vi "Error Handler Main.vi"(8 "Error In":errorcluster) -> ()   [LabVIEW 2014]
uses:
  <vilib>/Platform/TimedLoop/XDataNode/timing_clust.ctl
  <vilib>/Platform/TimedLoop/XDataNode/nitl_modes.ctl
  <vilib>/Platform/TimedLoop/XDataNode/wakeup.ctl
  <vilib>/Utility/error.llb/DialogType.ctl
  Stop Button/SubVI/Get Stop Button Status.vi
  <vilib>/platform/TimedLoop/XDataNode/XDataNode.xnode
  <vilib>/Platform/TimedLoop/XDataNode/XDNodeRunTimeDep.lvlib
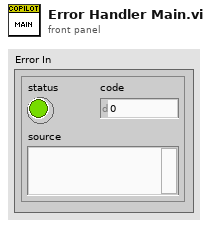
[diagram p1: front panel]
types:
  T1 = typedef "XDNodeRunTimeDep.lvlib/timing_clust.ctl" = cluster{"Expected End [f-1]":u64, "Actual End [f-1]":u64, "Finished Late? [f-1]":bool, "Expected End [i-1]":u64, "Actual End [i-1]":u64, "Finished Late? [i-1]":bool, "Expected Start [i]":u64, "Actual Start [i]":u64, "Expected Start [f]":u64, "Actual Start [f]":u64, "Source Name":string, "Structure Name":string, "Period":i64, "Deadline":i64, "Offset":i64, "Start":i64, "Priority":i32, "Timeout":i32, "Mode":T2, "Wakeup Reason":T3, "Error":errorcluster, "Source Type":string, "Secondary Source Type":string, "Global End Time":u64, "Global Start Time":u64, "Frame Duration":u64, "Iteration Duration":u64, "Assigned CPU":i32, "I/O Scan Engine Mode":u32}
  T2 = typedef "XDNodeRunTimeDep.lvlib/nitl_modes.ctl" = enum32{"No Change", "Process missed periods, maintain original phase", "Discard missed periods, maintain original phase", "Process missed periods, ignore original phase", "Discard missed periods, ignore original phase"}
  T3 = typedef "XDNodeRunTimeDep.lvlib/wakeup.ctl" = enum32{"Normal", "Aborted", "Asynchronous wakeup", "Timing source error", "Timed loop error", "Timeout"}
  T4 = typedef "DialogType.ctl" = u16
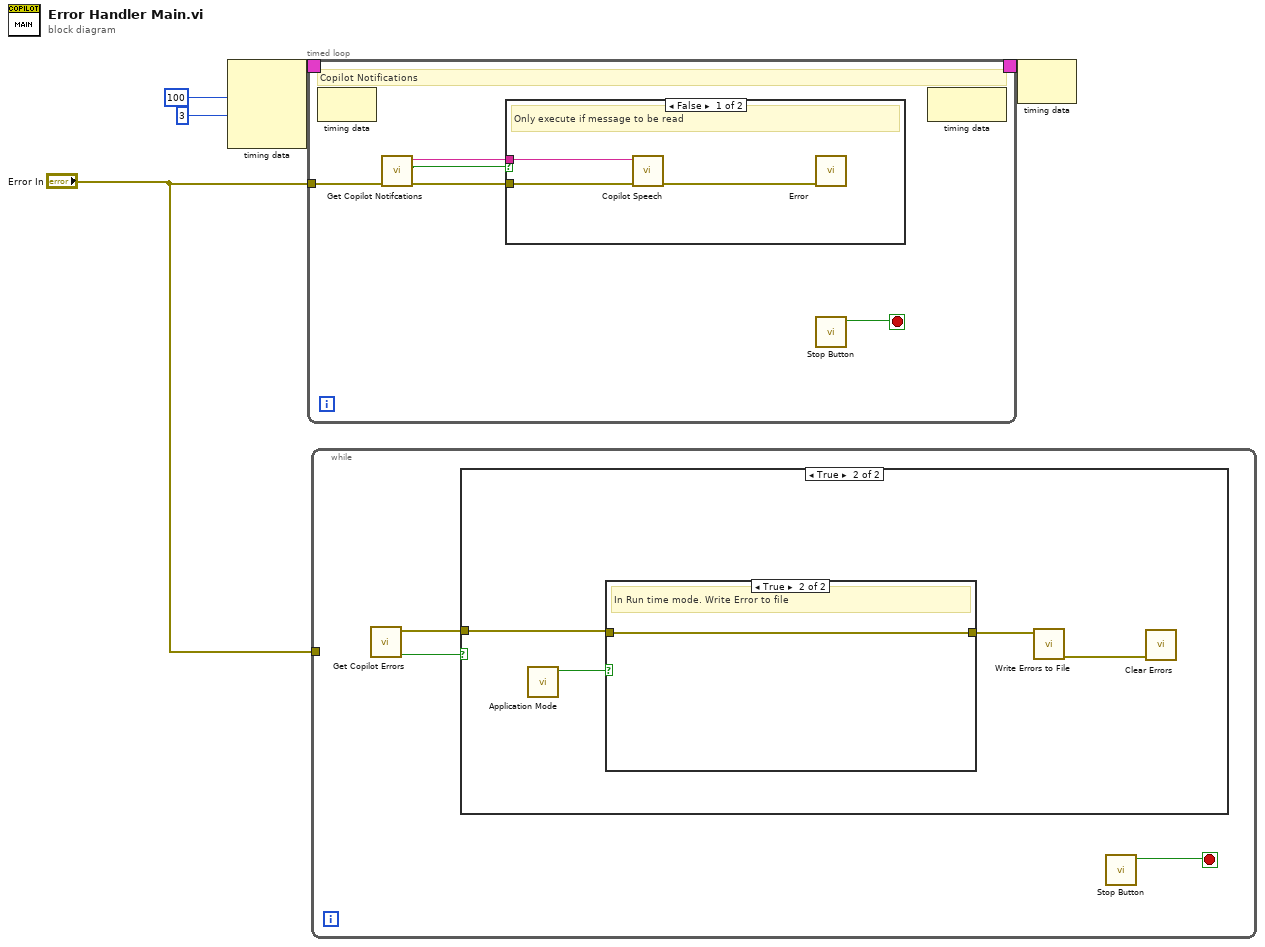
[diagram p0: block diagram]
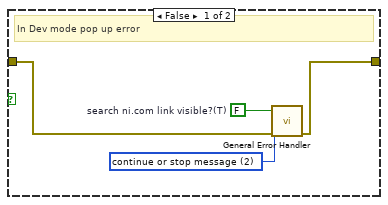
[diagram p3: hidden frame]
diagram:
  n1 = node-c288(i64 100 ("Period"), 3 ("Priority")) -> (w5:T1)  [unwired: 2 in]
  n2 = timed-loop {
    timing: w5 -> [_]
    timing-out: [_] -> w4
    tunnel: "Error In" -> [w7]
    stop <- w8 stop-if-true
    # "Copilot Notifications"
    n3 = node-c288() -> ()  [unwired: 1 in, 1 out]
    n4 = call "Get Copilot Notifcations.vi"("Error In"=w7) -> ("error out"=w9:errorcluster, "timed out?"=w6:bool, "Notification"=w10:string)  [unwired: 8 in]
    n5 = case shown="False" w6 {
      tunnel: w10 -> [w13 _]
      tunnel: w9 -> [w12 _]
      frame False {
        # "Only execute if message to be read"
        n6 = call "Copilot Speech.vi"("error in (no error)"=w12, "TEXT TO BE SPOKEN"=w13) -> ("error out"=w11:errorcluster)  [unwired: 9 in]
        n7 = call "Error.vi"("Error In"=w11) -> ()  [unwired: 10 in, 1 out]
      }
      frame True {
      }
    }
    n8 = call-poly "Stop Button.vi"() -> ("Stop ButtonOut"=w8:bool)  [unwired: 10 in, 1 out]
    n9 = node-c288() -> ()  [unwired: 1 in, 1 out]
  }
  n10 = while {
    tunnel: "Error In" -> [_]
    stop <- w18 stop-if-true
    n11 = call "Get Copilot Errors.vi"() -> ("Errors Pressent?"=w16:bool, "Error Out"=w17:errorcluster)  [unwired: 10 in]
    n12 = case shown="True" w16 {
      tunnel: w17 -> [_ w20]
      frame False {
      }
      frame True {
        n13 = call "Application Mode.vi"() -> ("Run Time Mode?"=w22:bool)  [unwired: 10 in, 1 out]
        n14 = case shown="True" w22 {
          tunnel: w20 -> [w26 w27]
          tunnel: [w23 w27] -> w21
          frame False {
            w24 = T4 2 items=["no dialog", "OK message", "continue or stop message", "OK message + warnings", "continue/stop + warnings"] ("type of dialog (OK msg:1)")
            w25 = FALSE  # search ni.com link visible?(T)
            # "In Dev mode pop up error"
            n15 = call <vilib>:"General Error Handler.vi"("search ni.com link visible?(T)"=w25, "type of dialog (OK msg:1)"=w24, "error in (no error)"=w26) -> ("error out"=w23:errorcluster)  [unwired: 8 in, 4 out]
          }
          frame True {
            # "In Run time mode. Write Error to file"
          }
        }
        n16 = call "Write Errors to File.vi"("Ground Station Errors"=w21) -> ("Error Out"=w19:errorcluster)  [unwired: 10 in]
        n17 = call <vilib>:"Clear Errors.vi"("error in (no error)"=w19) -> ()  [unwired: 5 in, 2 out]
      }
    }
    n18 = call-poly "Stop Button.vi"() -> ("Stop ButtonOut"=w18:bool)  [unwired: 10 in, 1 out]
  }
  n19 = node-c288(w4) -> ()  [unwired: 1 out]
